vi "Global P.vi"() -> ()   [LabVIEW 2015]
panel:
  out "P":cluster{"1":dbl, " S2":dbl}
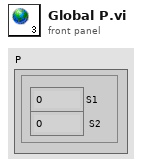
[diagram p1: front panel]
diagram:
